vi "Send Show GUI Message.vi"(6 "Show GUI Options":T1, 7 "High Priority (F)":bool, 8 "error in (no error)":errorcluster, 11 "Module in":refnum<class "Module.lvclass">) -> (0 "error out":errorcluster, 3 "Module out":refnum<class "Module.lvclass">)   [LabVIEW 2020, in "Volatus.lvlib" / "Module.lvclass"]
uses:
  Module.lvclass
  Module.lvclass/Module.ctl
  Volatus.lvlib
  Show GUI Options.ctl
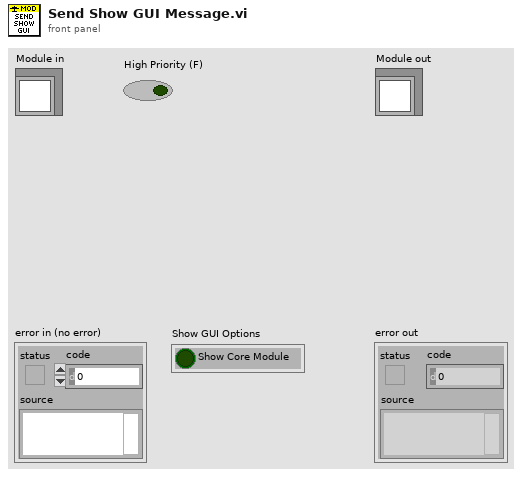
[diagram p1: front panel]
types:
  T1 = typedef "Volatus.lvlib/Show GUI Options.ctl" = cluster{"Show Core Module":bool}
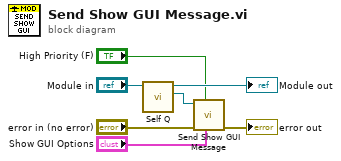
[diagram p0: block diagram]
diagram:
  n1 = call "Self Q.vi"("Module in"="Module in") -> ("Self Q"=w5:refnum<class "MessageQ.lvclass">, "Module out"=→"Module out":refnum<class "Module.lvclass">)  [unwired: 9 in]
  n2 = call "Send Show GUI Message.vi"("Show GUI Options"="Show GUI Options", "High Priority (F)"="High Priority (F)", "error in (no error)"="error in (no error)", "MessageQ"=w5) -> ("error out"=→"error out":errorcluster)  [unwired: 7 in]
